vi "instrumentProperties_model.vi"(5 "error in (no error)":errorcluster, 7 "spectrIdx":u16) -> (15 "model":string, 19 "error out":errorcluster)   [LabVIEW 2010, in "OSA.lvclass"]
doc: "Lower level init routine."
uses:
  OSA.lvclass
  _dll/LVLib/FTSLib.lvlib
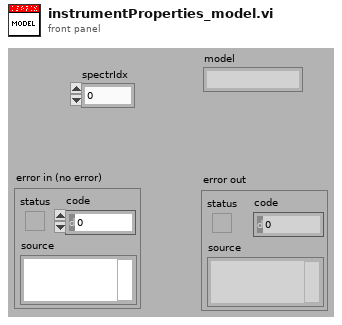
[diagram p1: front panel]
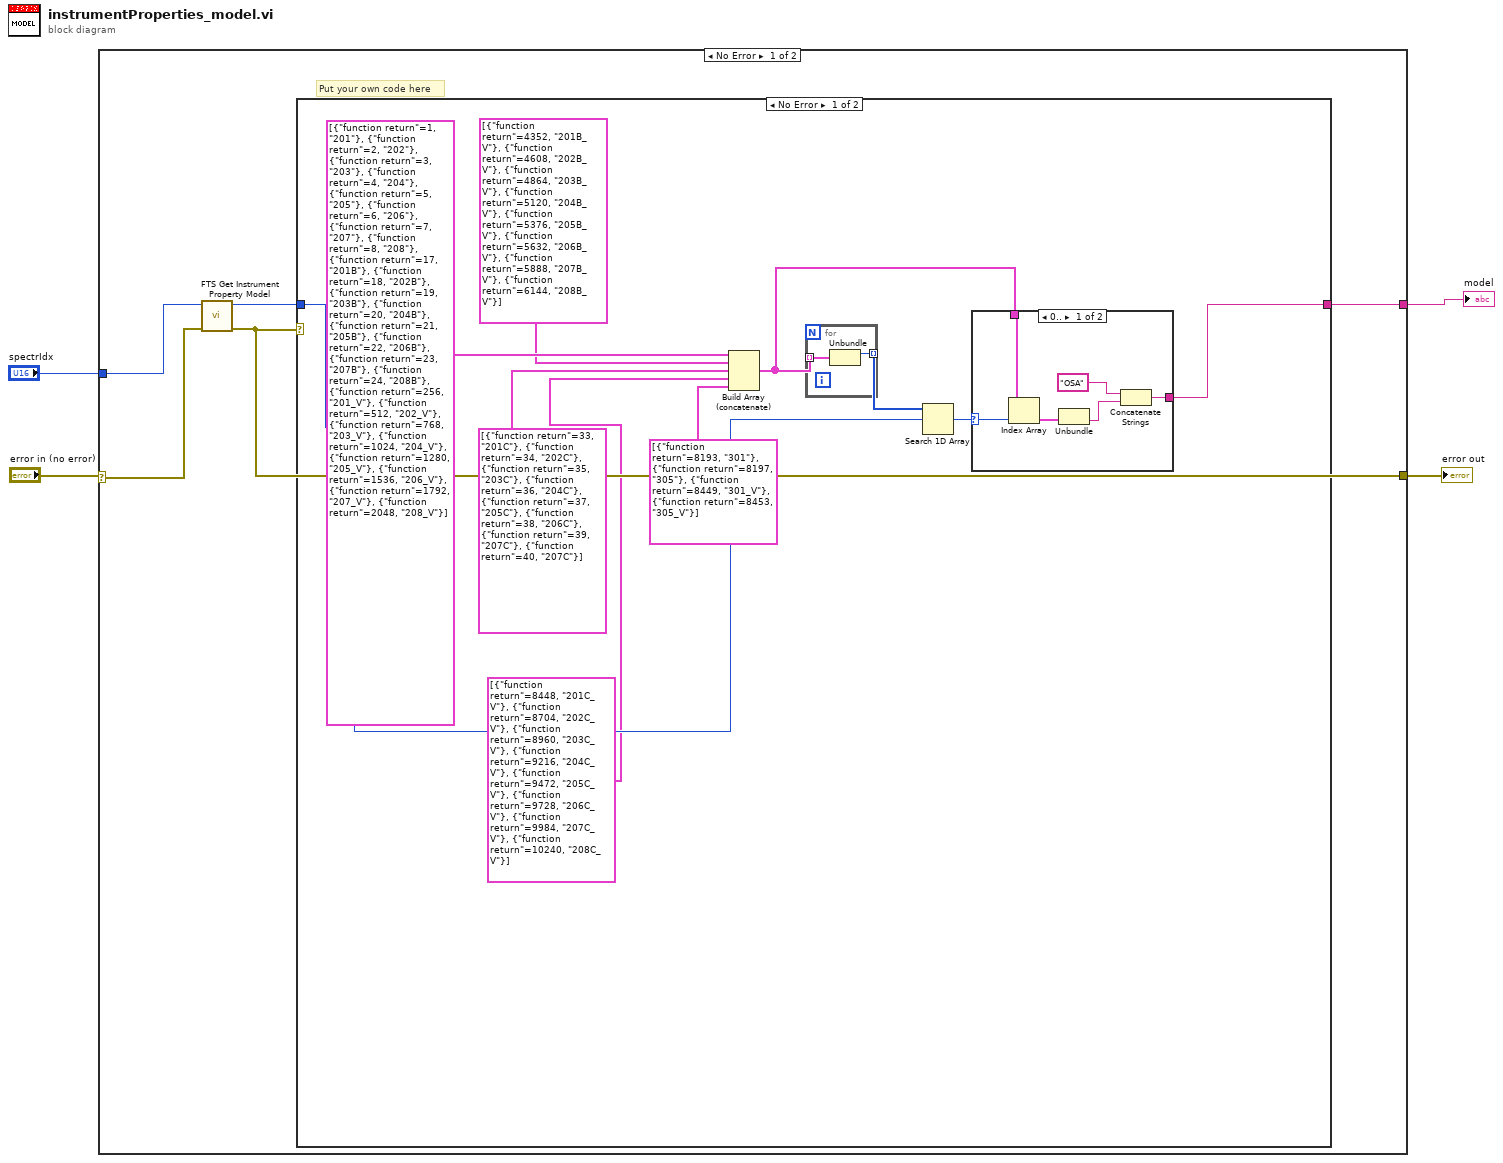
[diagram p0: block diagram]
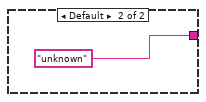
[diagram p2: hidden frame]
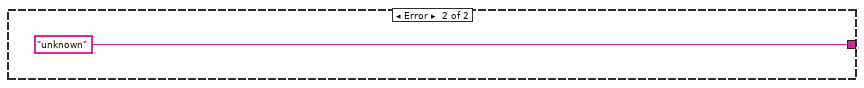
[diagram p3: hidden frame]
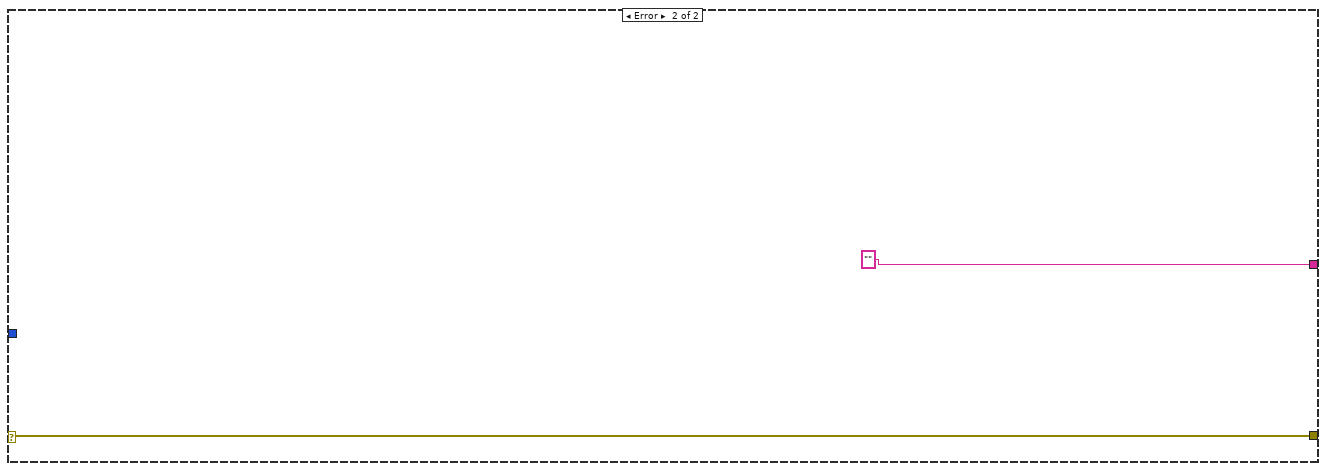
[diagram p4: hidden frame]
diagram:
  n1 = case shown="No Error" "error in (no error)" {
    selector: "error in (no error)" -> [w8 w31]
    tunnel: [w5 w31] -> w4
    tunnel: "spectrIdx" -> [w9 _]
    tunnel: [w7 ""] -> w1
    frame No Error {
      # "Put your own code here"
      n2 = call "FTS Get Instrument Property Model.vi"("error in (no error)"=w8, "specIndex"=w9) -> ("error out"=w5:errorcluster, "function return"=w6:u16)  [unwired: 8 in]
      n3 = case shown="No Error" w5 {
        tunnel: [w13 "unknown" ("model string")] -> w7
        tunnel: w6 -> [w14 _]
        frame No Error {
          n4 = Build Array (concatenate)(cluster{"function return":u16, string}[] [{"function return"=1, "201"}, {"function return"=2, "202"}, {"function return"=3, "203"}, {"function return"=4, "204"}, {"function return"=5, "205"}, {"function return"=6, "206"}, {"function return"=7, "207"}, {"function return"=8, "208"}, {"function return"=17, "201B"}, {"function return"=18, "202B"}, {"function return"=19, "203B"}, {"function return"=20, "204B"}, {"function return"=21, "205B"}, {"function return"=22, "206B"}, {"function return"=23, "207B"}, {"function return"=24, "208B"}, {"function return"=256, "201_V"}, {"function return"=512, "202_V"}, {"function return"=768, "203_V"}, {"function return"=1024, "204_V"}, {"function return"=1280, "205_V"}, {"function return"=1536, "206_V"}, {"function return"=1792, "207_V"}, {"function return"=2048, "208_V"}], cluster{"function return":u16, string}[] [{"function return"=4352, "201B_V"}, {"function return"=4608, "202B_V"}, {"function return"=4864, "203B_V"}, {"function return"=5120, "204B_V"}, {"function return"=5376, "205B_V"}, {"function return"=5632, "206B_V"}, {"function return"=5888, "207B_V"}, {"function return"=6144, "208B_V"}], cluster{"function return":u16, string}[] [{"function return"=33, "201C"}, {"function return"=34, "202C"}, {"function return"=35, "203C"}, {"function return"=36, "204C"}, {"function return"=37, "205C"}, {"function return"=38, "206C"}, {"function return"=39, "207C"}, {"function return"=40, "207C"}], cluster{"function return":u16, string}[] [{"function return"=8448, "201C_V"}, {"function return"=8704, "202C_V"}, {"function return"=8960, "203C_V"}, {"function return"=9216, "204C_V"}, {"function return"=9472, "205C_V"}, {"function return"=9728, "206C_V"}, {"function return"=9984, "207C_V"}, {"function return"=10240, "208C_V"}], cluster{"function return":u16, string}[] [{"function return"=8193, "301"}, {"function return"=8197, "305"}, {"function return"=8449, "301_V"}, {"function return"=8453, "305_V"}]) -> (w15:cluster{"function return":u16, string}[])
          n5 = for {
            tunnel: w15 -> [w28] mode=indexing
            tunnel: [w27] -> w19 mode=indexing
            n6 = Unbundle(w28) -> ("function return"=w27:u16)  [unwired: 1 out]
          }
          n7 = Search 1D Array(1D array=w19, element=w14) -> (index of element=w18:i32)  [unwired: 1 in]
          n8 = case shown="0.." w18 {
            selector: w18 -> [w24 _]
            tunnel: w15 -> [w25 _]
            tunnel: [w20 "unknown"] -> w13
            frame 0.. {
              n9 = Index Array(array=w25, index=w24) -> (element=w23:cluster{"function return":u16, string})
              n10 = Unbundle(w23) -> (w21:string)  [unwired: 1 out]
              n11 = Concatenate Strings("OSA", w21) -> (w20:string)
            }
            frame Default {
            }
          }
        }
        frame Error {
        }
      }
    }
    frame Error {
      # "Error"
    }
  }
  "error out" <- w4
  "model" <- w1
